vi "RF Rec Read and Write AXI-4 Stream.vi"(0 "port clock":refnum<k21>, 1 "rx 0.sfp fifo":refnum<k21>="Ch0 Rx to SFP0", 2 "rx 1.sfp fifo":refnum<k21>="Ch1 Rx to SFP0", 5 "TX niInstr AXI4-Stream Reader FXP64x1 v1 FPGA out":refnum<class "niInstr AXI4-Stream Writer FXP64x1 v1 FPGA.lvclass">, 7 "RX niInstr AXI4-Stream Reader FXP64x1 v1 FPGA out":refnum<class "niInstr AXI4-Stream Reader FXP64x1 v1 FPGA.lvclass">, 9 "port debug CLIP resources":T1, 11 "port debug info":refnum<k21>, 12 "tx 0.sfp fifo":refnum<k21>="SFP0 to Ch0 Tx", 13 "tx 1.sfp fifo":refnum<k21>="SFP0 to Ch1 Tx") -> ()   [LabVIEW 2018]
uses:
  <instrlib>/_niInstr/CLIP Adapters/v1/FPGA/AXI4-Stream/Writer FXP64x1/niInstr AXI4-Stream Writer FXP64x1 v1 FPGA.lvclass
  C:/Program Files (x86)/National Instruments/LabVIEW 2018/instr.lib/_niInstr/CLIP Adapters/v1/FPGA/AXI4-Stream/Writer/niInstr AXI4-Stream Writer v1 FPGA.lvclass
  <instrlib>/_niInstr/CLIP Adapters/v1/FPGA/AXI4-Stream/Reader FXP64x1/niInstr AXI4-Stream Reader FXP64x1 v1 FPGA.lvclass
  C:/Program Files (x86)/National Instruments/LabVIEW 2018/instr.lib/_niInstr/CLIP Adapters/v1/FPGA/AXI4-Stream/Reader/niInstr AXI4-Stream Reader v1 FPGA.lvclass
  <vilib>/Platform/TimedLoop/XDataNode/timing_clust.ctl
  <vilib>/Platform/TimedLoop/XDataNode/nitl_modes.ctl
  <vilib>/Platform/TimedLoop/XDataNode/wakeup.ctl
  <vilib>/rvi/Emulation/niFpgaSctlEmulationGetInTimedLoop.vi
  <vilib>/rvi/Emulation/niFpgaEmulationReportErrorSimple.vi
  <vilib>/rvi/Emulation/niFpgaGetClockAttributes.vi
  <vilib>/rvi/Emulation/niFpgaCriticalErrorInLSC.vi
  <vilib>/rvi/DataTransferAndStorage/Container/Common/niFpgaContainerExecOnDevCompGetState.vi
  <vilib>/rvi/Emulation/niFpgaEmulationIsFPGAContextNoSignature.vi
  <vilib>/rvi/DataTransferAndStorage/Container/Common/niFpgaContainerGetUniqueNameForEmu.vi
  <vilib>/rvi/Memory/Memory_Emulation/niFpgaMemoryEmulationCacheClearOnFirstRun.vi
  <vilib>/rvi/Memory/Memory_Emulation/nirvimemoryEmulationManagerCache_MakeExclusive.vi
  <vilib>/rvi/Memory/Memory_Emulation/niFpgaMemoryEmulationValidateCache.vi
  <vilib>/rvi/Memory/Memory_Emulation/nirvimemoryEmulationManagerCache_InsertValue.vi
  <vilib>/Utility/error.llb/Clear Errors.vi
  <vilib>/rvi/Memory/Memory_Emulation/nirvimemoryEmulationManagerCache_ReleaseExclusive.vi
  <vilib>/rvi/Memory/Memory_Emulation/nirvimemoryEmulationManagerCache_GetValue.vi
  <vilib>/rvi/Memory/Memory_Emulation/nirvimemoryEmulationManagerCache_SetValue.vi
  <vilib>/rvi/Emulation/niFpgaProcessEmulError.vi
  <vilib>/rvi/errors/niFpgaSetErrorForExecOnDevCompSimple.vi
  <vilib>/rvi/eio/common/nirviEmuReportErrorAndStop.vi
  <vilib>/rvi/FIFO/Fifo_Resource/nirvififoEmulationSetSize.vi
  <vilib>/rvi/FIFO/Fifo_Resource/nirviFifoEmulationQueueMgr.vi
  <instcachedir>/0/nirviFifoEmulationQueueMgr_E5CAEC123FF24DC58D834DCA3CDAA9B5.lvgen/nirviFifoEmulationQueueMgr_E5CAEC123FF24DC58D834DCA3CDAA9B5_000.vi
  <vilib>/rvi/FIFO/Fifo_Resource/nirvififoEmulationDetermineInputValidOut.vi
  <vilib>/rvi/FIFO/Fifo_Resource/nirvififoEmulationCreateLock.vi
  <vilib>/rvi/FIFO/Fifo_Resource/nirvififoEmulationObtainLock.vi
  <vilib>/rvi/FIFO/Fifo_Resource/nirvififoEmulationReleaseLock.vi
  <vilib>/rvi/occurrence/nirviWaitOnOccurrenceBase.vi
  <vilib>/rvi/errors/nirviReportUnexpectedCaseInternalError.vi
  <vilib>/rvi/errors/nirviReportUnexpectedCaseInternalError (U32).vi
  <vilib>/rvi/interface/RandomDataEmulation/niFpgaRandomDataHandleErrors.vi
  <vilib>/Platform/TimedLoop/XDataNode/XDataNode.xnode
  <vilib>/rvi/DataTransferAndStorage/Container/XNode/niFpgaContainer.xnode
  <vilib>/rvi/DataTransferAndStorage/Register/Emulation/niFpgaRegisterEmulationRefIn.vi
  <vilib>/rvi/FIFO/Fifo_Resource/niFpgaFifoEmulationRefIn.vi
  <vilib>/Platform/TimedLoop/XDataNode/XDNodeRunTimeDep.lvlib
  <instrlib>/_niInstr/CLIP Adapters/v1/FPGA/AXI4-Stream/Writer/niInstr AXI4-Stream Writer v1 FPGA.lvclass
  <instrlib>/_niInstr/CLIP Adapters/v1/FPGA/AXI4-Stream/Reader/niInstr AXI4-Stream Reader v1 FPGA.lvclass
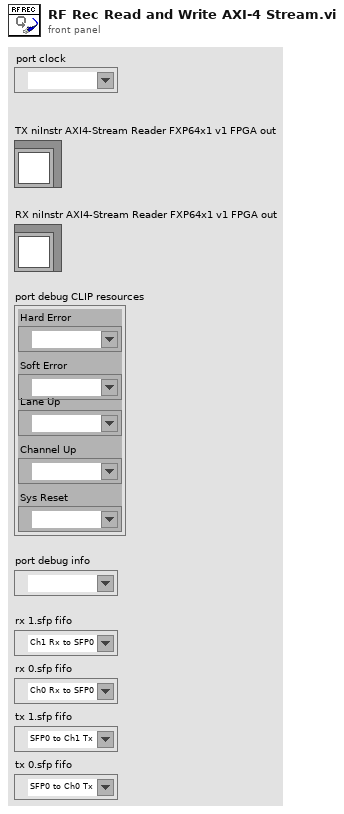
[diagram p1: front panel]
types:
  T1 = cluster{"Hard Error":refnum<k21>, "Soft Error":refnum<k21>, "Lane Up":refnum<k21>, "Channel Up":refnum<k21>, "Sys Reset":refnum<k21>}
  T2 = typedef "XDNodeRunTimeDep.lvlib/timing_clust.ctl" = cluster{"Expected End [f-1]":u64, "Actual End [f-1]":u64, "Finished Late? [f-1]":bool, "Expected End [i-1]":u64, "Actual End [i-1]":u64, "Finished Late? [i-1]":bool, "Expected Start [i]":u64, "Actual Start [i]":u64, "Expected Start [f]":u64, "Actual Start [f]":u64, "Source Name":string, "Structure Name":string, "Period":i64, "Deadline":i64, "Offset":i64, "Start":i64, "Priority":i32, "Timeout":i32, "Mode":T3, "Wakeup Reason":T4, "Error":errorcluster, "Source Type":string, "Secondary Source Type":string, "Global End Time":u64, "Global Start Time":u64, "Frame Duration":u64, "Iteration Duration":u64, "Assigned CPU":i32, "I/O Scan Engine Mode":u32}
  T3 = typedef "XDNodeRunTimeDep.lvlib/nitl_modes.ctl" = enum32{"No Change", "Process missed periods, maintain original phase", "Discard missed periods, maintain original phase", "Process missed periods, ignore original phase", "Discard missed periods, ignore original phase"}
  T4 = typedef "XDNodeRunTimeDep.lvlib/wakeup.ctl" = enum32{"Normal", "Aborted", "Asynchronous wakeup", "Timing source error", "Timed loop error", "Timeout"}
  T5 = typedef "RF Rec Port Debug Info.ctl" = cluster{"hard error":bool, "soft error":bool, "lane up":bool, "channel up":bool, "sys reset":bool}
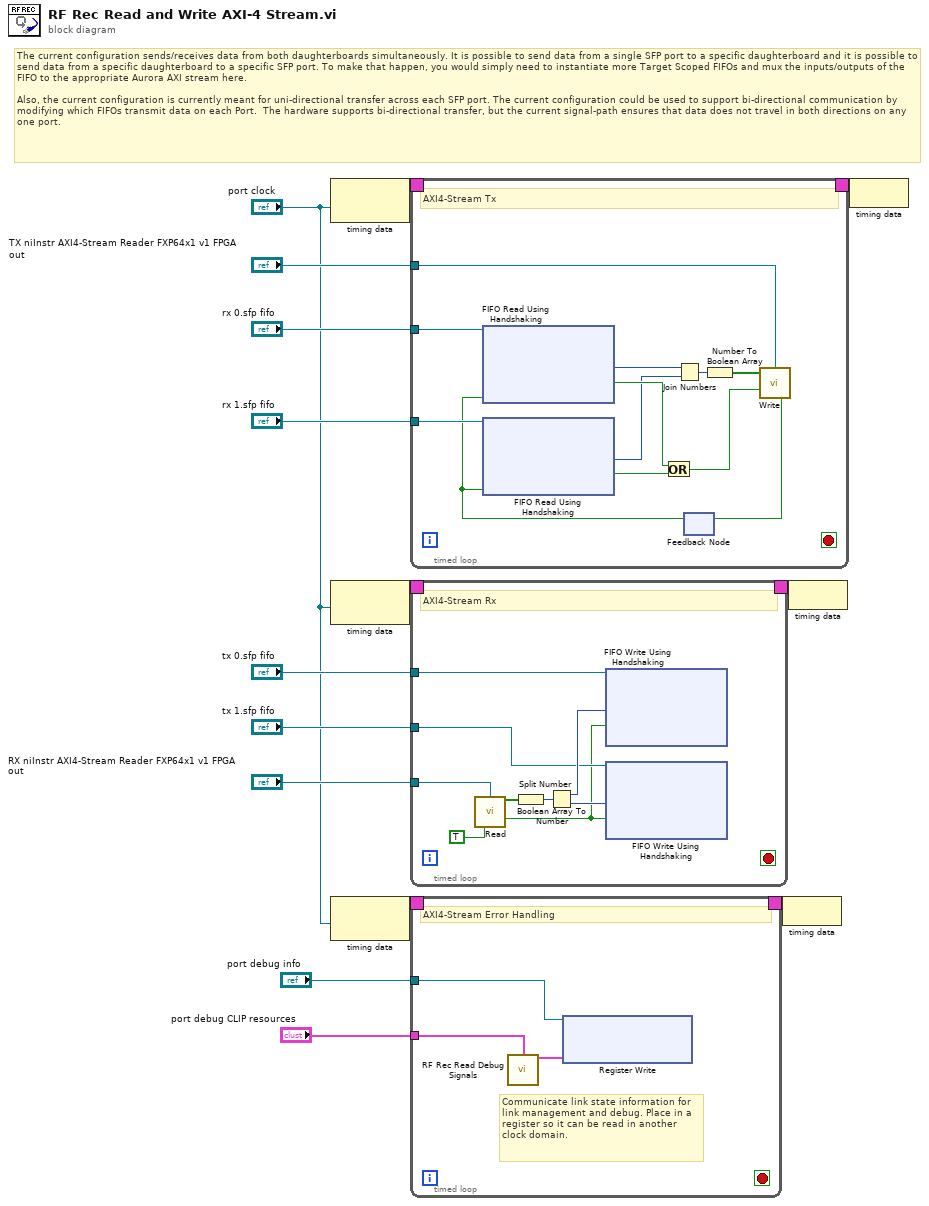
[diagram p0: block diagram]
diagram:
  # "The current configuration sends/receives data from both daughterboards simultaneously. It is possible to send data from a single SFP port to a specific daughterboard and it is possible to send data from a specific daughterboard to a specific SFP port. To make that happen, you would simply need to instantiate more Target Scoped FIFOs and mux the inputs/outputs of the FIFO to the appropriate Aurora AXI stream here. \n\nAlso, the current configuration is currently meant for uni-directional transfer across each SFP port. The current configuration could be used to support bi-directional communication by modifying which FIFOs transmit data on each Port.  The hardware supports bi-directional transfer, but the current signal-path ensures that data does not travel in both directions on any one port."
  n1 = node-c288("port clock") -> (w15:T2)
  n2 = node-c288("port clock") -> (w6:T2)
  n3 = node-c288("port clock") -> (w10:T2)
  n4 = timed-loop "Timed Loop" {
    timing: w15 -> [_]
    timing-out: [_] -> w14
    tunnel: "TX niInstr AXI4-Stream Reader FXP64x1 v1 FPGA out" -> [w24]
    tunnel: "rx 1.sfp fifo" -> [w23]
    tunnel: "rx 0.sfp fifo" -> [w22]
    stop <- _ stop-if-true
    # "AXI4-Stream Tx"
    n5 = feedback #1() -> (w16:bool)  [unwired: 1 in]
    n6 = xnode "FIFO Read Using Handshaking"("Ready for Output"=w16, "FIFO In"=w22) -> ("Element"=w18:u32, "Output Valid"=w21:bool)  [unwired: 1 out]
    n7 = xnode "FIFO Read Using Handshaking"("Ready for Output"=w16, "FIFO In"=w23) -> ("Element"=w17:u32, "Output Valid"=w20:bool)  [unwired: 1 out]
    n8 = Or(x=w21, y=w20) -> (x .or. y?=w19:bool)
    n9 = Join Numbers(hi=w18, lo=w17) -> ((hi.lo)=w25:u64)
    n10 = Number To Boolean Array(number=w25) -> (Boolean array=w26:bool[])
    n11 = call <instrlib>:"Write.vi"("tdata"=w26, "niInstr AXI4-Stream Writer v1 FPGA in"=w24, "input valid"=w19) -> ("ready for input"=w27:bool)  [unwired: 12 in]
    n12 = feedback-in #1(w27) -> ()
  }
  n13 = timed-loop "Timed Loop" {
    timing: w6 -> [_]
    timing-out: [_] -> w5
    tunnel: "RX niInstr AXI4-Stream Reader FXP64x1 v1 FPGA out" -> [w37]
    tunnel: "tx 0.sfp fifo" -> [w35]
    tunnel: "tx 1.sfp fifo" -> [w33]
    stop <- _ stop-if-true
    # "AXI4-Stream Rx"
    n14 = call <instrlib>:"Read.vi"("niInstr AXI4-Stream Reader v1 FPGA in"=w37, "ready for output"=TRUE) -> ("tdata"=w38:bool[], "output valid"=w31:bool)  [unwired: 8 in, 4 out]
    n15 = Boolean Array To Number(Boolean array=w38) -> (number=w36:u64)
    n16 = Split Number(x=w36) -> (hi(x)=w34:u32, lo(x)=w32:u32)
    n17 = xnode "FIFO Write Using Handshaking"("Element"=w34, "Input Valid"=w31, "FIFO In"=w35) -> ()  [unwired: 2 out]
    n18 = xnode "FIFO Write Using Handshaking"("Element"=w32, "Input Valid"=w31, "FIFO In"=w33) -> ()  [unwired: 2 out]
  }
  n19 = timed-loop {
    timing: w10 -> [_]
    timing-out: [_] -> w9
    tunnel: "port debug info" -> [w41]
    tunnel: "port debug CLIP resources" -> [w42]
    stop <- _ stop-if-true
    # "Communicate link state information for link management and debug. Place in a register so it can be read in another clock domain."
    # "AXI4-Stream Error Handling"
    n20 = call "RF Rec Read Debug Signals.vi"("Debug CLIP Resources"=w42) -> ("port debug info"=w43:T5)  [unwired: 14 in]
    n21 = xnode ("Register Write")("Data"=w43, "Register In"=w41) -> ()  [unwired: 1 out]
  }
  n22 = node-c288(w9) -> ()
  n23 = node-c288(w5) -> ()
  n24 = node-c288(w14) -> ()
